vi "update floor ceiling array.vi"(10 "Game Parameters":T3, 11 "Arrays and Heights":T1={"Score Array"=[], "Lowest high score"=0.0, "Score"=0.0, "Ceiling"=0.0, "Floor"=0.0, "Ceiling Array"=[], "Floor array"=[], "Helicopter height"=0.0, "Helicopter array"=[], "Fuel"=0.0, "Fuel array"=[], "fuel counter"=0, "obstacle counter"=0, "Obstacle array"=[], "helicopter v_0"=0.0, "helicopter a_0"=0.0, "Obstacle height"=300.0}) -> (3 "Arrays and Heights":T1={"Score Array"=[], "Lowest high score"=0.0, "Score"=0.0, "Ceiling"=0.0, "Floor"=0.0, "Ceiling Array"=[], "Floor array"=[], "Helicopter height"=0.0, "Helicopter array"=[], "Fuel"=300.0, "Fuel array"=[], "fuel counter"=0, "obstacle counter"=0, "Obstacle array"=[], "helicopter v_0"=0.0, "helicopter a_0"=0.0, "Obstacle height"=300.0})   [LabVIEW 2017]
uses:
  controls/game parameters.ctl
  controls/arrays and heights.ctl
  controls/scores.ctl
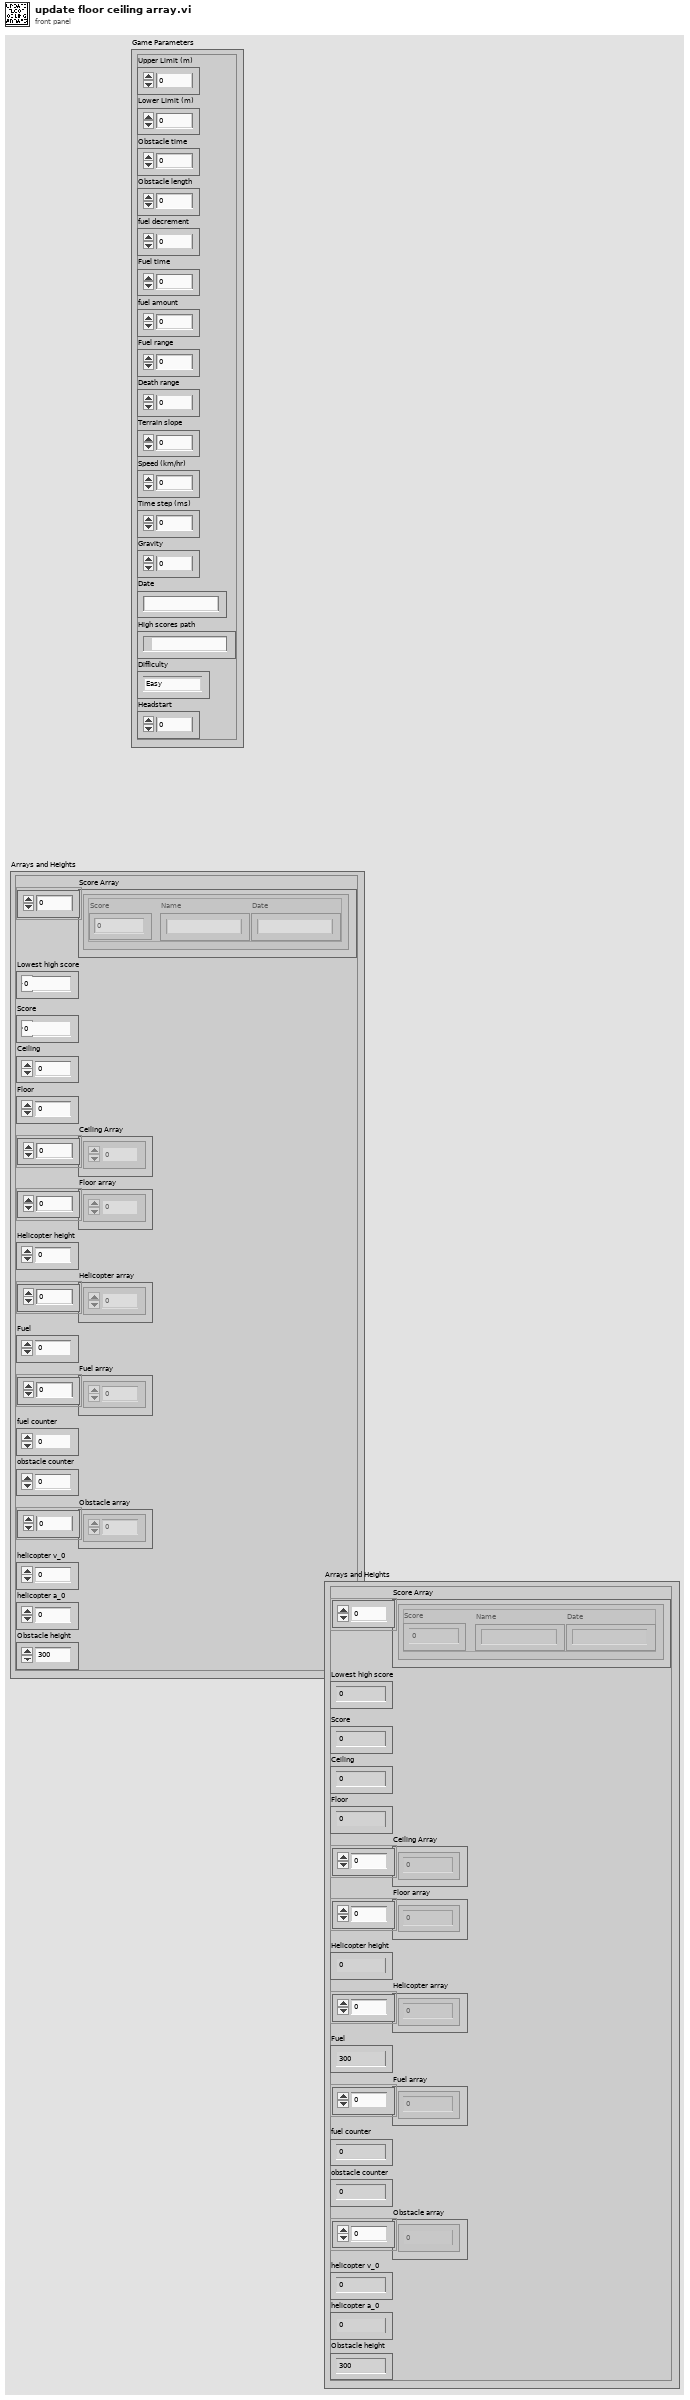
[diagram p1: front panel]
types:
  T1 = typedef "arrays and heights.ctl" = cluster{"Score Array":T2[], "Lowest high score":dbl, "Score":dbl, "Ceiling":dbl, "Floor":dbl, "Ceiling Array":dbl[], "Floor array":dbl[], "Helicopter height":dbl, "Helicopter array":dbl[], "Fuel":dbl, "Fuel array":dbl[], "fuel counter":i32, "obstacle counter":i32, "Obstacle array":dbl[], "helicopter v_0":dbl, "helicopter a_0":dbl, "Obstacle height":dbl}
  T2 = typedef "scores.ctl" = cluster{"Score":dbl, "Name":string, "Date":string}
  T3 = typedef "game parameters.ctl" = cluster{"Upper Limit (m)":dbl, "Lower Limit (m)":dbl, "Obstacle time":dbl, "Obstacle length":dbl, "fuel decrement":dbl, "Fuel time":dbl, "fuel amount":dbl, "Fuel range":i32, "Death range":i32, "Terrain slope":dbl, "Speed (km/hr)":dbl, "Time step (ms)":u32, "Gravity":dbl, "Date":string, "High scores path":path, "Difficulty":enum16{"Easy", "Normal", "Hard"}, "Headstart":u32}
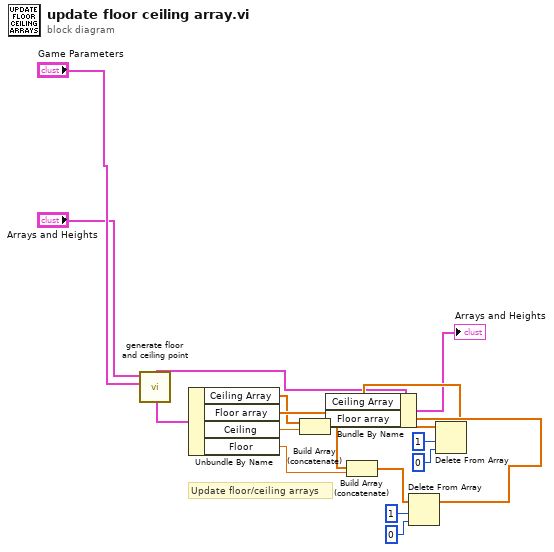
[diagram p0: block diagram]
diagram:
  # "Update floor/ceiling arrays"
  n1 = call "generate floor and ceiling point.vi"("Game Parameters"="Game Parameters", "Arrays and Heights"="Arrays and Heights") -> ("Arrays and values"=w13:T1)  [unwired: 9 in]
  n2 = Unbundle By Name(w13) -> ("Ceiling Array"=w8:dbl[], "Floor array"=w9:dbl[], "Ceiling"=w11:dbl, "Floor"=w12:dbl)
  n3 = Build Array (concatenate)(w8, w11) -> (w7:dbl[])
  n4 = Build Array (concatenate)(w9, w12) -> (w2:dbl[])
  n5 = Delete From Array(array=w2, length=1, index=0) -> (array with subset deleted=w15:dbl[])  [unwired: 1 out]
  n6 = Delete From Array(array=w7, length=1, index=0) -> (array with subset deleted=w14:dbl[])  [unwired: 1 out]
  n7 = Bundle By Name(cluster=w13, "Ceiling Array"=w14, "Floor array"=w15) -> (→"Arrays and Heights":T1)
